vi "Map RGB.vi"(6 "B":u8 format="%.0x", 8 "error in":errorcluster, 9 "G":u8 format="%.0x", 10 "R":u8 format="%.0x", 11 "Pixel Format":T1 {"Format" format="%.0x"; "Next Pointer" format="%.0x"; "Rmask" format="%.0x"; "Gmask" format="%.0x"; "Bmask" format="%.0x"; "Amask" format="%.0x"; "Palette Pointer" format="%.0x"}) -> (0 "error out":errorcluster, 3 "Colour":u32 format="%.0x")   [LabVIEW 2015, in "LibSDL2.lvlib"]
uses:
  LibSDL2.lvlib
  Controls/Pixel Formal.ctl
  DLL/SDL2.dll
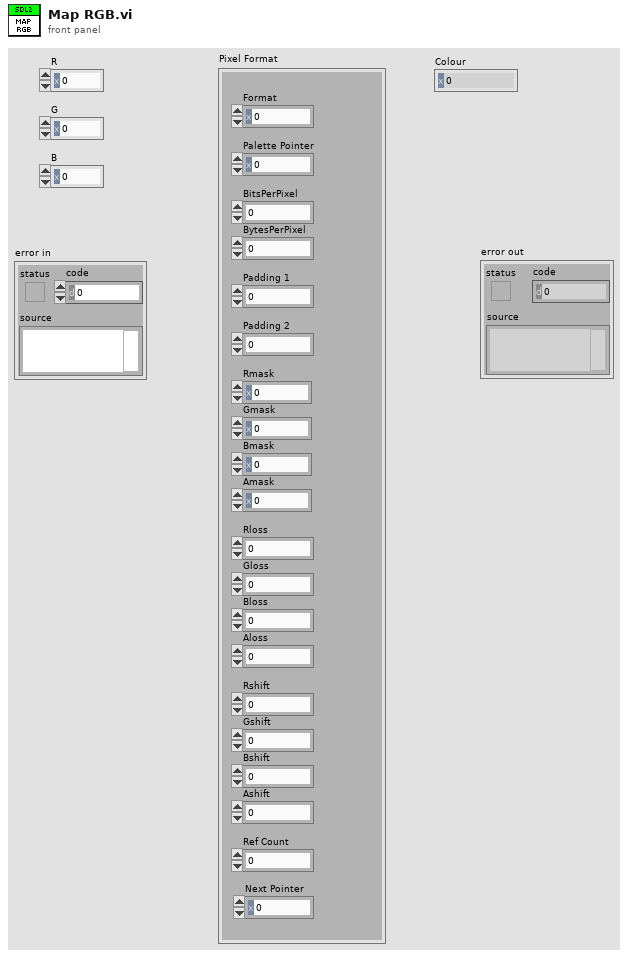
[diagram p1: front panel]
types:
  T1 = typedef "LibSDL2.lvlib/Pixel Formal.ctl" = cluster{"Format":u32, "Palette Pointer":u32, "BitsPerPixel":u8, "BytesPerPixel":u8, "Padding 1":u8, "Padding 2":u8, "Rmask":u32, "Gmask":u32, "Bmask":u32, "Amask":u32, "Rloss":u8, "Gloss":u8, "Bloss":u8, "Aloss":u8, "Rshift":u8, "Gshift":u8, "Bshift":u8, "Ashift":u8, "Ref Count":i32, "Next Pointer":u32}
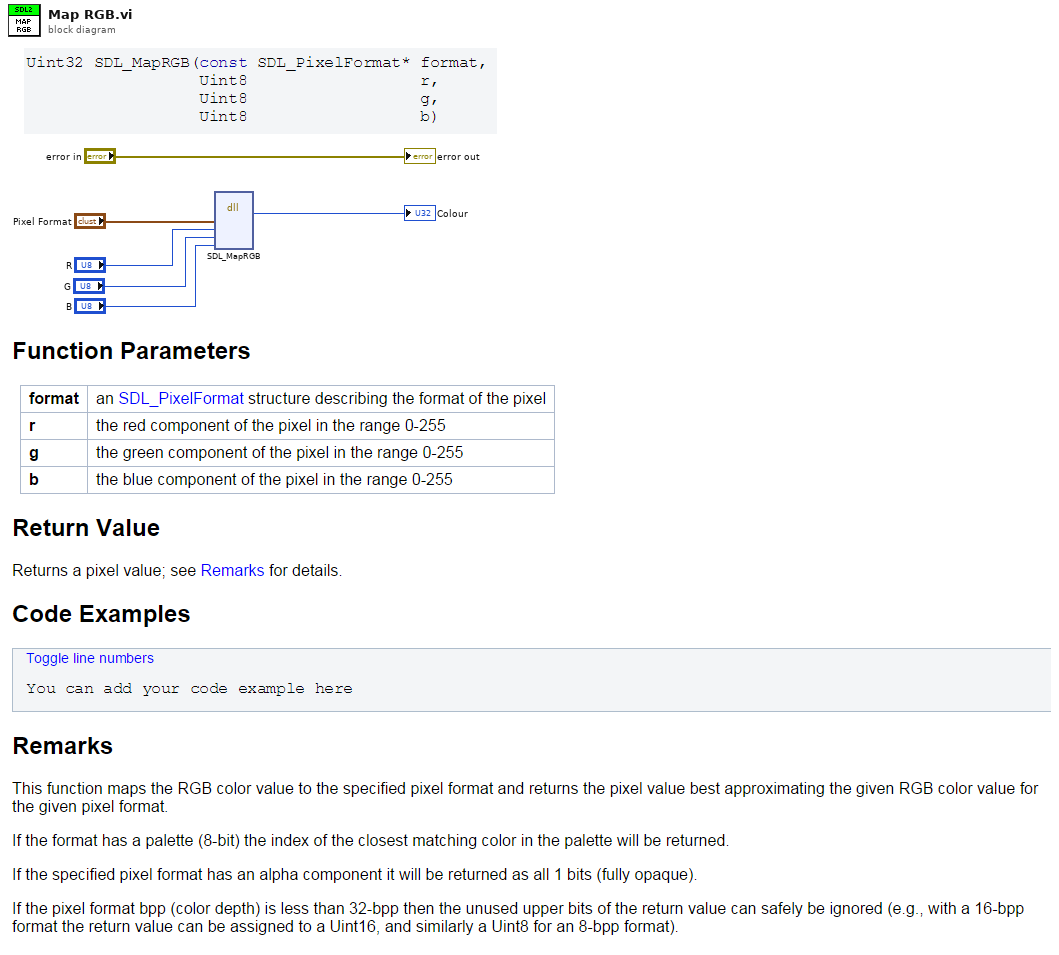
[diagram p0: block diagram]
diagram:
  n1 = dll-call lib="C:/dev/PGS/LabSDL2/Source/Libraries/LibSDL2 Wrapper/DLL/SDL2.dll" fn="SDL_MapRGB"("format"="Pixel Format", "r"="R", "g"="G", "b"="B") -> ("return type"=→"Colour":u32)  [unwired: 7 in, 2 out]
  "error out" <- "error in"
